vi "GenerateIEDevModeDiagnosticsCode.vi"(8 "error in (no error)":errorcluster) -> (3 "Diagnostics (u8)":u8)   [LabVIEW 2021]
doc: "Create an 8 bit diagnostics code that is used by downstream automation.\n\nBit 0: NIIconEditor\nBit 1: lv_icon.lvlibp\nBit 2: lv_IconEditor.lvlib \nBit 3: lv_icon.vi\nBit 4: lv_icon.vit \nBit 5: SAMPLE_lv_icon.vi \nBit 6: LabVIEW Icon API \nBit 7: All non-fatal paths"
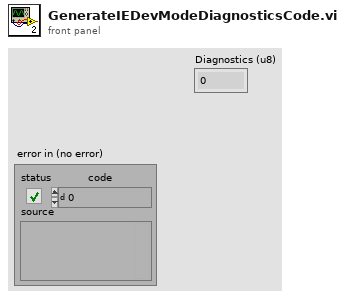
[diagram p1: front panel]
types:
  T1 = cluster{"NIIconEditor":bool, "lv_icon.lvlibp":bool, "lv_IconEditor.lvlib":bool, "lv_icon.vi":bool, "lv_icon.vit":bool, "SAMPLE_lv_icon.vi":bool, "LabVIEW Icon API":bool, "All non-fatal paths":bool}
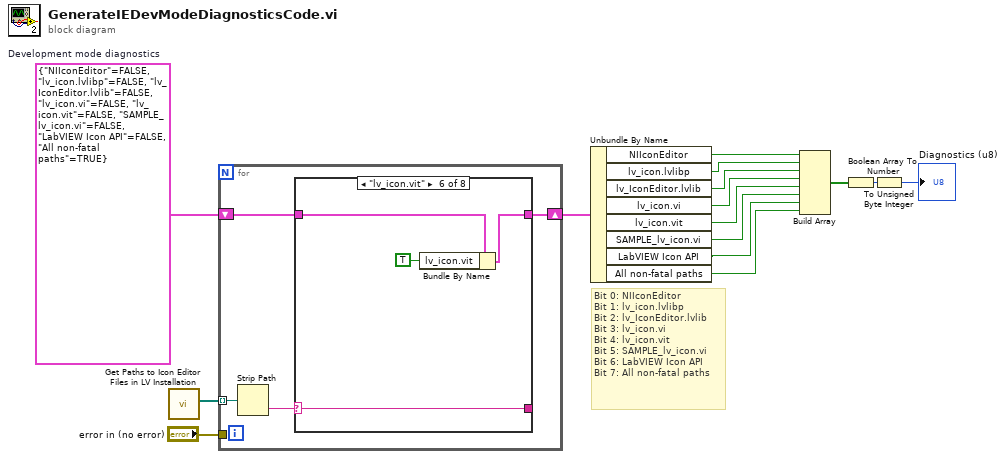
[diagram p0: block diagram]
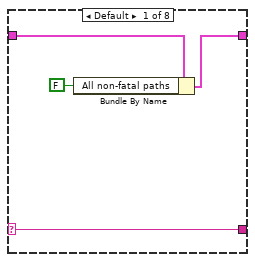
[diagram p2: hidden frame]
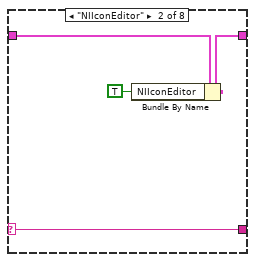
[diagram p3: hidden frame]
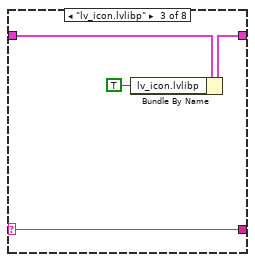
[diagram p4: hidden frame]
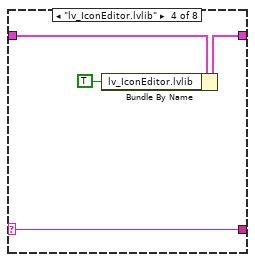
[diagram p5: hidden frame]
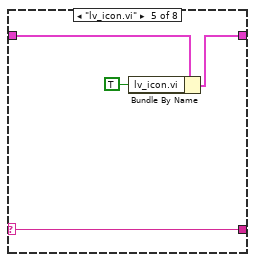
[diagram p6: hidden frame]
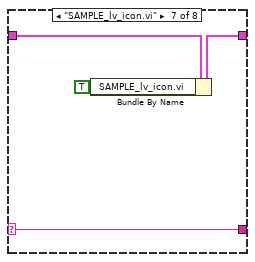
[diagram p7: hidden frame]
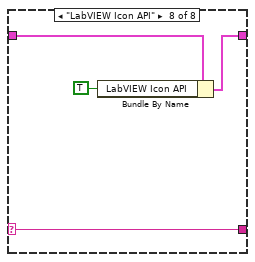
[diagram p8: hidden frame]
diagram:
  w14 = T1 {"NIIconEditor"=FALSE, "lv_icon.lvlibp"=FALSE, "lv_IconEditor.lvlib"=FALSE, "lv_icon.vi"=FALSE, "lv_icon.vit"=FALSE, "SAMPLE_lv_icon.vi"=FALSE, "LabVIEW Icon API"=FALSE, "All non-fatal paths"=TRUE}  # Development mode diagnostics
  # "Bit 0: NIIconEditor\nBit 1: lv_icon.lvlibp\nBit 2: lv_IconEditor.lvlib \nBit 3: lv_icon.vi\nBit 4: lv_icon.vit \nBit 5: SAMPLE_lv_icon.vi \nBit 6: LabVIEW Icon API \nBit 7: All non-fatal paths"
  n1 = call "Get Paths to Icon Editor Files in LV Installation.vi"() -> ("relative paths"=w15:path[])  [unwired: 10 in, 1 out]
  n2 = for {
    tunnel: w15 -> [w19] mode=indexing
    shift-right: [w16] -> w13
    shift-left: w14 -> [w17]
    tunnel: "error in (no error)" -> [_]
    n3 = Strip Path(path=w19) -> (name=w18:string)  [unwired: 1 out]
    n4 = case shown="\"lv_icon.vit\"" w18 {
      selector: w18 -> [w23 w27 w31 w35 w39 w43 w47 w51]
      tunnel: [w23 w27 w31 w35 w39 w43 w47 w51] -> _
      tunnel: w17 -> [w22 w26 w30 w34 w38 w42 w46 w50]
      tunnel: [w21 w25 w29 w33 w37 w41 w45 w49] -> w16
      frame Default {
        n5 = Bundle By Name(cluster=w22, "All non-fatal paths"=FALSE ("Unhandled path(s)")) -> (w21:T1)
      }
      frame "NIIconEditor" {
        n6 = Bundle By Name(cluster=w26, "NIIconEditor"=TRUE) -> (w25:T1)
      }
      frame "lv_icon.lvlibp" {
        n7 = Bundle By Name(cluster=w30, "lv_icon.lvlibp"=TRUE) -> (w29:T1)
      }
      frame "lv_IconEditor.lvlib" {
        n8 = Bundle By Name(cluster=w34, "lv_IconEditor.lvlib"=TRUE) -> (w33:T1)
      }
      frame "lv_icon.vi" {
        n9 = Bundle By Name(cluster=w38, "lv_icon.vi"=TRUE) -> (w37:T1)
      }
      frame "lv_icon.vit" {
        n10 = Bundle By Name(cluster=w42, "lv_icon.vit"=TRUE) -> (w41:T1)
      }
      frame "SAMPLE_lv_icon.vi" {
        n11 = Bundle By Name(cluster=w46, "SAMPLE_lv_icon.vi"=TRUE ("lv_icon.vit")) -> (w45:T1)
      }
      frame "LabVIEW Icon API" {
        n12 = Bundle By Name(cluster=w50, "LabVIEW Icon API"=TRUE) -> (w49:T1)
      }
    }
  }
  n13 = Unbundle By Name(w13) -> ("NIIconEditor"=w12:bool, "lv_icon.lvlibp"=w11:bool, "lv_IconEditor.lvlib"=w10:bool, "lv_icon.vi"=w9:bool, "lv_icon.vit"=w8:bool, "SAMPLE_lv_icon.vi"=w7:bool, "LabVIEW Icon API"=w6:bool, "All non-fatal paths"=w5:bool)
  n14 = Build Array(w12, w11, w10, w9, w8, w7, w6, w5) -> (w4:bool[])
  n15 = Boolean Array To Number(Boolean array=w4) -> (number=w3:u32)
  n16 = To Unsigned Byte Integer(number=w3) -> (unsigned 8bit integer=→"Diagnostics (u8)":u8)
